vi "Msg.vi"(7 "jettl in":refnum<class "jettl.lvclass">, 11 "Update Queue Nested Msg Strategy in":refnum<class "Update Queue Nested Msg Strategy.lvclass">) -> (5 "jettl out":refnum<class "jettl.lvclass">)   [LabVIEW 2021, in "jettl.lvlib" / "Update Queue Nested.lvlib" / "Update Queue Nested Msg Strategy.lvclass"]
uses:
  Update Queue Nested Msg Strategy.lvclass
  jettl/jettl/jettl.lvclass
  Update Queue Nested/Update Queue Nested.lvclass
  Update Queue Nested Msg Strategy.lvclass/Update Queue Nested Msg Strategy.ctl
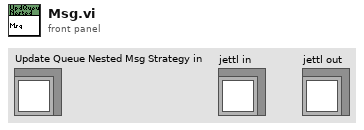
[diagram p1: front panel]
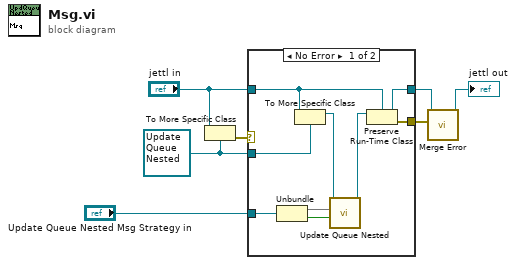
[diagram p0: block diagram]
diagram:
  w4 = refnum<class "Update Queue Nested.lvclass"> refnum ("Update Queue Nested.lvlib:Update Queue Nested.lvclass")
  n1 = To More Specific Class(target class=w4, reference="jettl in") -> (error out=w7:errorcluster)  [unwired: 1 in, 1 out]
  n2 = case shown="No Error" w7 {
    selector: w7 -> [_ w17]
    tunnel: [w14 w18] -> w5
    tunnel: "jettl in" -> [w15 w18]
    tunnel: w4 -> [w16 _]
    tunnel: [w13 w17] -> w6
    tunnel: "Update Queue Nested Msg Strategy in" -> [w10 _]
    frame No Error {
      n3 = Unbundle(w10) -> (w9:map{string, refnum<data-value>}, w8:bool)
      n4 = To More Specific Class(target class=w16, reference=w15) -> (specific class reference=w12:refnum<class "Update Queue Nested.lvclass">)  [unwired: 1 in, 1 out]
      n5 = call-dynamic "Update Queue Nested.vi"("Insert (T) or Remove (F)"=w8, "Queue Nested"=w9, "Update Queue Nested in"=w12) -> ("Update Queue Nested out"=w11:refnum<class "Update Queue Nested.lvclass">)  [unwired: 8 in]
      n6 = Preserve Run-Time Class(object in=w11, 2:w15) -> (object out=w14:refnum<class "jettl.lvclass">, error out=w13:errorcluster)  [unwired: 1 in]
    }
    frame Error {
    }
  }
  n7 = call-dynamic "Merge Error.vi"("Error"=w6, "jettl in"=w5) -> ("jettl out"=→"jettl out":refnum<class "jettl.lvclass">)  [unwired: 9 in]
